vi "Read TDMS Wavenames.vi"(8 "error in (no error)":errorcluster, 11 "path":path) -> (0 "error out":errorcluster, 2 "Wavenames":string[](array[string]), 3 "file path out":path)   [LabVIEW 2019, in "LV-Data.TDMS.lvclass"]
uses:
  LV-Data.TDMS.lvclass
panel:
  in  "Index (0)":i32
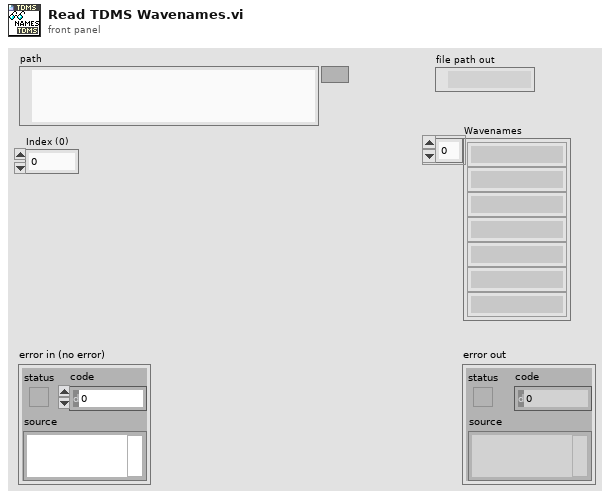
[diagram p1: front panel]
types:
  T1 = enum16{"open", "open or create", "create or replace", "create", "open (read-only)"}
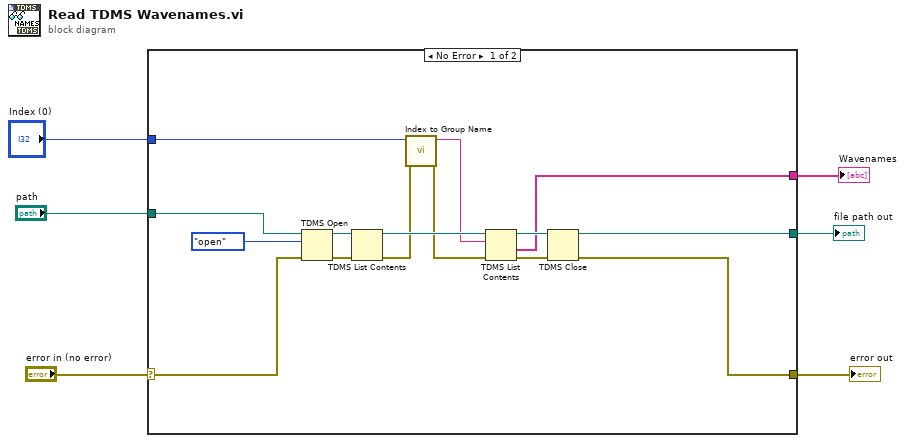
[diagram p0: block diagram]
diagram:
  n1 = case shown="No Error" "error in (no error)" {
    selector: "error in (no error)" -> [w16 w22]
    tunnel: [w20 w22] -> w5
    tunnel: "path" -> [w19 _]
    tunnel: [w15 _] -> w3
    tunnel: [w14 _] -> w2
    tunnel: "Index (0)" -> [w7 _]
    frame No Error {
      n2 = TDMS Open(8:w16, 10:T1."open" ("operation (0:open)"), 11:w19) -> (0:w11:errorcluster, 3:w13:refnum<k34>)  [unwired: 4 in]
      n3 = TDMS List Contents(4:w11, 7:w13) -> (0:w9:errorcluster, 3:w12:refnum<k34>)  [unwired: 1 in, 2 out]
      n4 = call "Index to Group Name.vi"("error in (no error)"=w9, "Append Index"=w7) -> ("error out"=w8:errorcluster, "group name in (Untitled)"=w10:string)  [unwired: 8 in]
      n5 = TDMS List Contents(4:w8, 6:w10, 7:w12) -> (0:w18:errorcluster, 1:w15:string[], 3:w17:refnum<k34>)  [unwired: 1 out]
      n6 = TDMS Close(8:w18, 11:w17) -> (0:w20:errorcluster, 3:w14:path)
    }
    frame Error {
    }
  }
  "error out" <- w5
  "Wavenames" <- w3
  "file path out" <- w2
